vi "Util_Set FP Size Position.vi"(8 "error in (no error)":errorcluster, 9 "Origin":T1, 10 "Front Panel Window:Panel Bounds":T2, 11 "Operation":enum16{"Get Postion", "Set Position"}(ring)) -> (0 "error out":errorcluster, 1 "Origin":T1, 2 "Front Panel Window:Panel Bounds":T2)   [LabVIEW 2013]
uses:
  <vilib>/Utility/miscctls.llb/LVRectTypeDef.ctl
  <vilib>/Utility/miscctls.llb/LVPointTypeDef.ctl
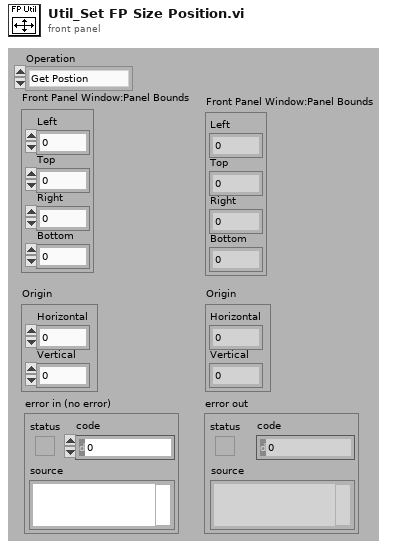
[diagram p1: front panel]
types:
  T1 = typedef "LVPointTypeDef.ctl" = cluster{"Horizontal":i16, "Vertical":i16}
  T2 = typedef "LVRectTypeDef.ctl" = cluster{"Left":i16, "Top":i16, "Right":i16, "Bottom":i16}
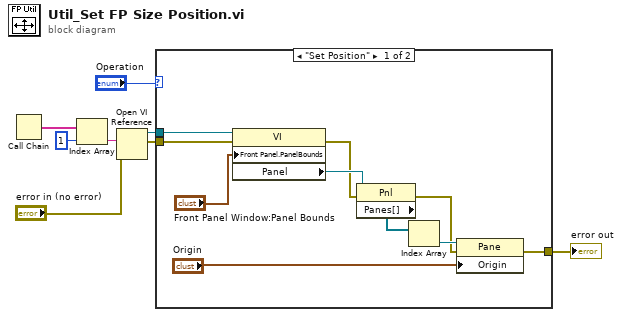
[diagram p0: block diagram]
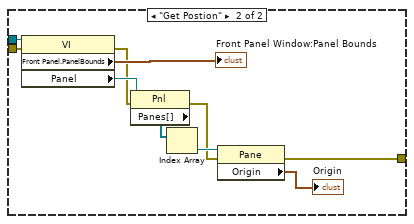
[diagram p2: hidden frame]
diagram:
  n1 = Call Chain() -> (call chain=w5:string[])
  n2 = Index Array(array=w5, index=1) -> (element=w3:string)
  n3 = Open VI Reference(vi path=w3, error in (no error)="error in (no error)") -> (vi reference=w6:refnum<vi>, error out=w8:errorcluster)  [unwired: 4 in]
  n4 = case shown="\"Set Position\"" "Operation" {
    tunnel: w6 -> [w13 w25]
    tunnel: w8 -> [w12 w24]
    tunnel: [w9 w19] -> w1
    frame "Set Position" {
      n5 = property class="VI"(reference=w13, error in=w12, "Front Panel.PanelBounds"="Front Panel Window:Panel Bounds") -> (error out=w11:errorcluster, "Panel"=w18:refnum<vi>)  [unwired: 1 out]
      n6 = property class="Pnl"(reference=w18, error in=w11) -> (error out=w10:errorcluster, "Panes[]"=w14:refnum<vi>[])  [unwired: 1 out]
      n7 = Index Array(array=w14) -> (element=w15:refnum<vi>)  [unwired: 1 in]
      n8 = property class="Pane"(reference=w15, error in=w10, "Origin"="Origin") -> (error out=w9:errorcluster)  [unwired: 1 out]
    }
    frame "Get Postion" {
      n9 = property class="VI"(reference=w25, error in=w24) -> (error out=w21:errorcluster, "Front Panel.PanelBounds"=→"Front Panel Window:Panel Bounds":T2, "Panel"=w28:refnum<vi>)  [unwired: 1 out]
      n10 = property class="Pnl"(reference=w28, error in=w21) -> (error out=w20:errorcluster, "Panes[]"=w26:refnum<vi>[])  [unwired: 1 out]
      n11 = Index Array(array=w26) -> (element=w27:refnum<vi>)  [unwired: 1 in]
      n12 = property class="Pane"(reference=w27, error in=w20) -> (error out=w19:errorcluster, "Origin"=→"Origin":T1)  [unwired: 1 out]
    }
  }
  "error out" <- w1
